vi "micro path.vi"(11 "Config":string) -> (3 "appended path":path)   [LabVIEW 2020]
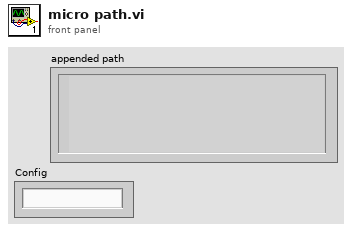
[diagram p1: front panel]
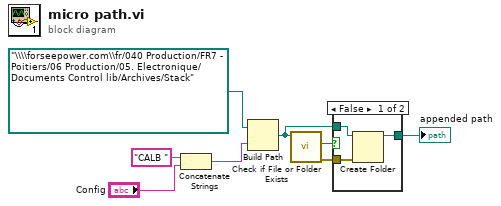
[diagram p0: block diagram]
diagram:
  n1 = Concatenate Strings("CALB " ("string"), "Config") -> (w2:string)
  n2 = Build Path ("Composer un chemin")(base path=path "\\\\forseepower.com\\fr/040 Production/FR7 - Poitiers/06 Production/05. Electronique/Documents Control lib/Archives/Stack" ("chemin de la cible (utiliser une boîte de dialogue)"), name or relative path=w2) -> (appended path=w6:path)
  n3 = call <vilib>:"Check if File or Folder Exists.vi"("path"=w6) -> ("error out"=w4:errorcluster, "file or folder exists?"=w7:bool)  [unwired: 8 in, 1 out]
  n4 = case shown="False" w7 {
    tunnel: w4 -> [w11 _]
    tunnel: w6 -> [w10 w12]
    tunnel: [w9 w12] -> w5
    frame False {
      n5 = Create Folder ("Créer un dossier")(path (use dialog)=w10, error in=w11) -> (created path=w9:path)  [unwired: 1 in, 2 out]
    }
    frame True {
    }
  }
  "appended path" <- w5
